vi "ELVIS III v1.0 RPC App Ref.vi"() -> (2 "Lib Path":path=path "/usr/local/natinst/academic/lib/niElvisIIIHost", 3 "RPC Reference":refnum<vi>)   [LabVIEW 2021]
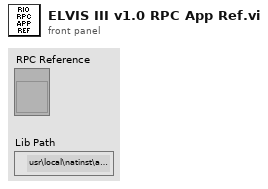
[diagram p1: front panel]
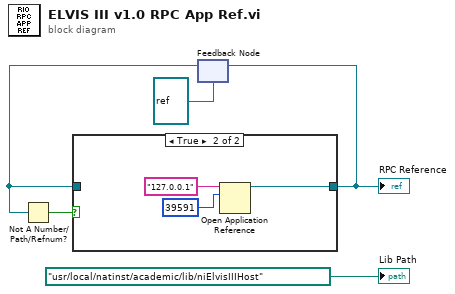
[diagram p0: block diagram]
diagram:
  n1 = feedback #1(refnum<vi> refnum ("application reference")) -> (w4:refnum<vi>)
  n2 = Not A Number/Path/Refnum?(number/path/refnum=w4) -> (NaN/Path/Refnum?=w3:bool)
  n3 = case shown="True" w3 {
    tunnel: [w6 w7] -> w5
    tunnel: w4 -> [w6 _]
    frame False {
    }
    frame True {
      n4 = Open Application Reference(10:u16 39591 ("port number or service name (3363)"), 11:"127.0.0.1" ("IP address")) -> (3:w7:refnum<vi>)  [unwired: 2 in, 1 out]
    }
  }
  "RPC Reference" <- w5
  n5 = feedback-in #1(w5) -> ()
  "Lib Path" <- path "/usr/local/natinst/academic/lib/niElvisIIIHost"
